vi "Measure Events (Non-40MHz).vi"(7 "settings.<user name>":T5, 8 "register bus":T3={"Speed"="Speed", "Crank Angle"="Crank Angle", "Cycle Angle"="Cycle Angle", "Crank Count"="Crank Count", "Cycle Count"="Cycle Count", "1.25 MHz Counter"="1.25 MHz Counter", "Crank Rollover"="Crank Rollover", "Cycle Rollover"="Cycle Rollover", "shared settings"={"start"=0.0, "stuck limit"=0.0}} {"shared settings"."start" format="%#.15g"}, 10 "event":bool) -> (2 "measured data":T2, 3 "status.<user name>":T1)   [LabVIEW 2013, in "Engine Simulation Toolkit.lvlib" / "ECU Event Timing.lvlib"]
doc: "Measures the characteristics of digital events (pulses) within a given angular position window. Combine this VI with 1 or more Event Capture.vi's to send event measurement data up to NI VeriStand.\n\n<b>settings.<user name></b> - settings for the component. NI VeriStand will set these values. Create a control for this input. Replace <user name> with the name you wish this component to display as inside NI VeriStand. Make this name consistent for all controls, indicators, for all VIs of this component.\n<b>event</b> - digital event (pulse) to measure. Can be active high or active low, NI VeriStand has a setting for configuring this.\n<b>register bus</b> - connect this input to the output of the initialize APU VI. This contains references to APU state variables like position and speed.\n\n<b>status.<user name></b> - output for the component. NI VeriStand will read these values. Create an indicator for this output. Replace <user name> with the name you wish this component to display as inside NI VeriStand. Make this name consistent for all controls, indicators, for all VIs of this component.\n<b>measured data</b> - event data to be wired to the Capture Event.vi"
uses:
  ECU Event Timing.lvlib
  Measure Settings.ctl
  APU/Register Bus.ctl
  APU/Shared Settings.ctl
  Measured Data.ctl
  Measure Output.ctl
  APU/APU.lvlib
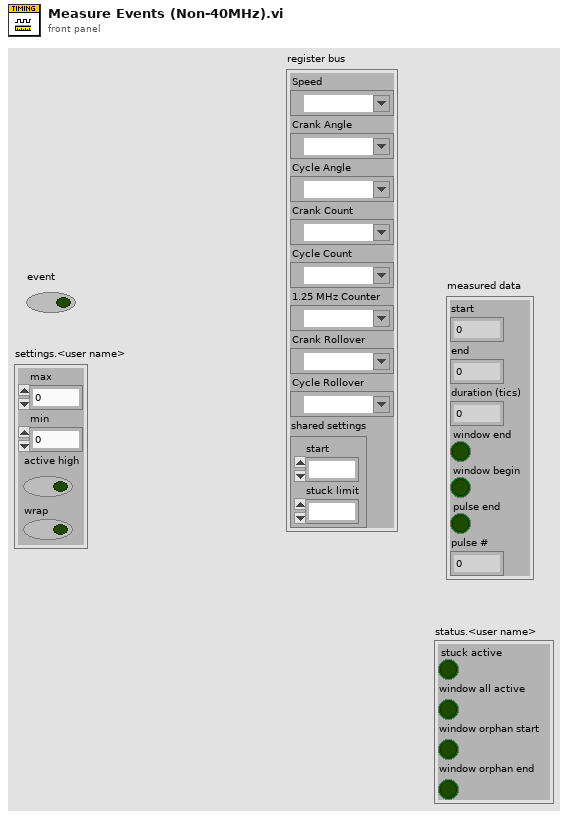
[diagram p1: front panel]
types:
  T1 = typedef "Engine Simulation Toolkit.lvlib/ECU Event Timing.lvlib/Measure Output.ctl" = cluster{"stuck active":bool, "window all active":bool, "window orphan start":bool, "window orphan end":bool}
  T2 = typedef "Engine Simulation Toolkit.lvlib/ECU Event Timing.lvlib/Measured Data.ctl" = cluster{"start":u16, "end":u16, "duration (tics)":fxp<+,18,18>, "window end":bool, "window begin":bool, "pulse end":bool, "pulse #":u8}
  T3 = typedef "Engine Simulation Toolkit.lvlib/APU.lvlib/Register Bus.ctl" = cluster{"Speed":refnum<k21>, "Crank Angle":refnum<k21>, "Cycle Angle":refnum<k21>, "Crank Count":refnum<k21>, "Cycle Count":refnum<k21>, "1.25 MHz Counter":refnum<k21>, "Crank Rollover":refnum<k21>, "Cycle Rollover":refnum<k21>, "shared settings":T4}
  T4 = typedef "Engine Simulation Toolkit.lvlib/APU.lvlib/Shared Settings.ctl" = cluster{"start":fxp<+,17,17>, "stuck limit":fxp<+,18,18>}
  T5 = typedef "Engine Simulation Toolkit.lvlib/ECU Event Timing.lvlib/Measure Settings.ctl" = cluster{"max":u16, "min":u16, "active high":bool, "wrap":bool}
  T6 = typedef "Engine Simulation Toolkit.lvlib/ECU Event Timing.lvlib/Windowed Event Data.ctl" = cluster{"end of window":bool, "begining of window":bool, "rising edge in window":bool, "falling edge in window":bool, "line active":bool, "1.25MHz tics since pulse started":fxp<+,18,18>, "cycle angle":u16, "stuck active":bool}
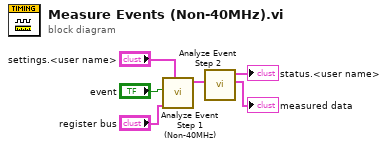
[diagram p0: block diagram]
diagram:
  n1 = call "Analyze Event Step 1 (Non-40MHz).vi"("measure settings.<user name>"="settings.<user name>", "register bus"="register bus", "event"="event") -> ("windowed event data"=w4:T6)  [unwired: 8 in]
  n2 = call "Analyze Event Step 2.vi"("windowed event data"=w4) -> ("measured data"=→"measured data":T2, "measure output.<user name>"=→"status.<user name>":T1)  [unwired: 9 in]
